vi "Set ITC LPF Needle Valve.vi"(8 "error in (no error)":errorcluster, 10 "Percentage Open (%)":dbl format="%#.2f", 11 "Instrument.Oxford1820 in":refnum<class "Instrument.OxfordVRM.lvclass">) -> (0 "error out":errorcluster, 2 "Response":string, 3 "Instrument.Oxford1820 out":refnum<class "Instrument.OxfordVRM.lvclass">)   [LabVIEW 2016, in "Instrument.OxfordVRM.lvclass"]
uses:
  Instrument.OxfordVRM.lvclass
  <instrlib>/Mercury iXX/Mercury iXX.lvlib
  <instrlib>/Mercury iXX/Public/Libraries/Lambda/Configuration/Set/Lambda Percentage Flow (Set).vi
  <instrlib>/Mercury iXX/Public/Libraries/Lambda.lvlib
  <instrlib>/Mercury iXX/Public/Libraries/Lambda/Open/Open Lambda Device.vi
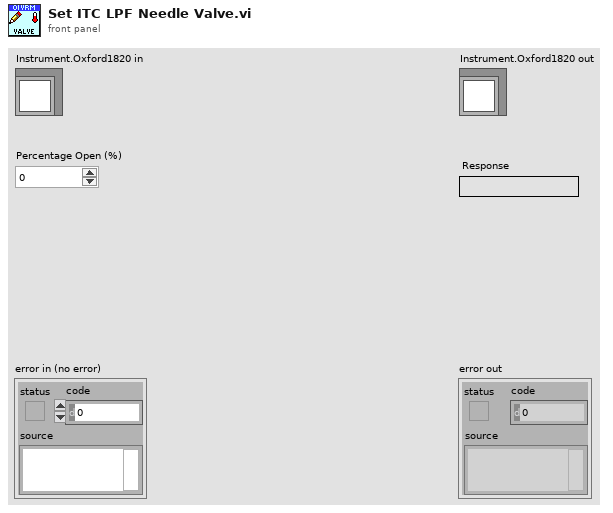
[diagram p1: front panel]
types:
  T1 = typedef "Mercury iXX.lvlib/Mercury Reference.ctl" = cluster{"Comms":refnum<visa-resource-name>, "Device ID":string[], "Comms Layer":T2, "Command":string, "Query reference":T3}
  T2 = typedef "Mercury iXX.lvlib/Comms Transport Layer.ctl" = enum16{"Ethernet TCP/IP", "USB", "ISOBus - RS-232", "GPIB"}
  T3 = typedef "Mercury iXX.lvlib/Query Dynamic Reference.ctl" = refnum<vi>
  T4 = typedef "Mercury iXX.lvlib/Response String.ctl" = string
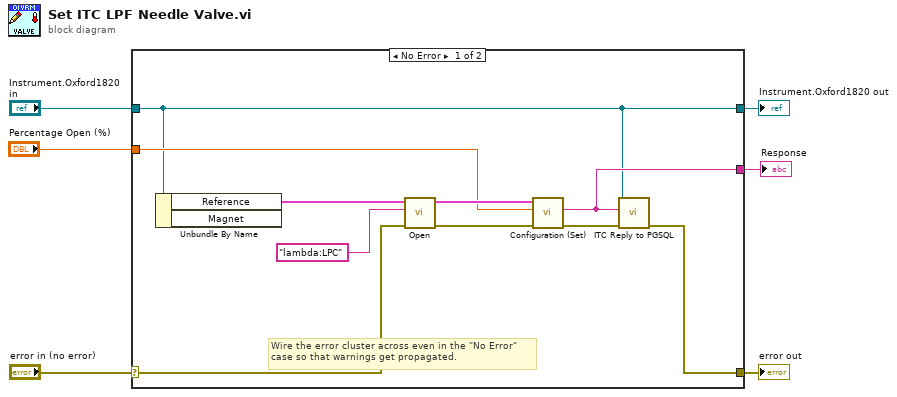
[diagram p0: block diagram]
diagram:
  n1 = case shown="No Error" "error in (no error)" {
    selector: "error in (no error)" -> [w14 w18]
    tunnel: [w9 w18] -> w5
    tunnel: [w7 w17] -> w3
    tunnel: "Instrument.Oxford1820 in" -> [w7 w17]
    tunnel: [w8 _] -> w2
    tunnel: "Percentage Open (%)" -> [w11 _]
    frame No Error {
      # "Wire the error cluster across even in the \"No Error\"\ncase so that warnings get propagated."
      n2 = Unbundle By Name(w7) -> ("Reference"=w15:T1)  [unwired: 1 out]
      n3 = call-poly <instrlib>:"Open.vi"("error in (no error)"=w14, "Device Identifier"="lambda:LPC", "Mercury Reference In"=w15) -> ("error out"=w13:errorcluster, "Mercury Reference Out"=w12:T1)  [unwired: 7 out]
      n4 = call-poly <instrlib>:"Configuration (Set).vi"("error in"=w13, "Percentage Open"=w11, "Mercury Reference In"=w12) -> ("error out"=w10:errorcluster, "Response"=w8:T4)  [unwired: 5 in, 2 out]
      n5 = call "ITC Reply to PGSQL.vi"("error in (no error)"=w10, "Response"=w8, "Instrument.1820 in"=w7) -> ("error out"=w9:errorcluster)  [unwired: 7 in, 1 out]
    }
    frame Error {
    }
  }
  "error out" <- w5
  "Instrument.Oxford1820 out" <- w3
  "Response" <- w2
